vi "SetTensionVelocity.vi"(8 "error in (no error)":errorcluster, 11 "Tapedrive_ESP301 in":refnum<class "Tapedrive_ESP301.lvclass">) -> (0 "error out":errorcluster, 3 "Tapedrive_ESP301 out":refnum<class "Tapedrive_ESP301.lvclass">)   [LabVIEW 2013, in "Tapedrive_ESP301.lvclass"]
uses:
  Tapedrive_ESP301.lvclass
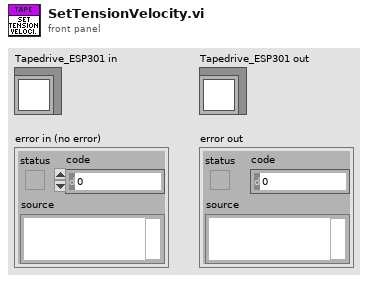
[diagram p1: front panel]
types:
  T1 = cluster{"Axis 1":cluster{"Value":dbl, "Min":dbl, "Max":dbl, "StepSize":dbl, "Tolerance":dbl, "ValueActual":dbl}, "Axis 2":cluster{"Value":dbl, "Min":dbl, "Max":dbl, "StepSize":dbl, "Tolerance":dbl, "ValueActual":dbl}}
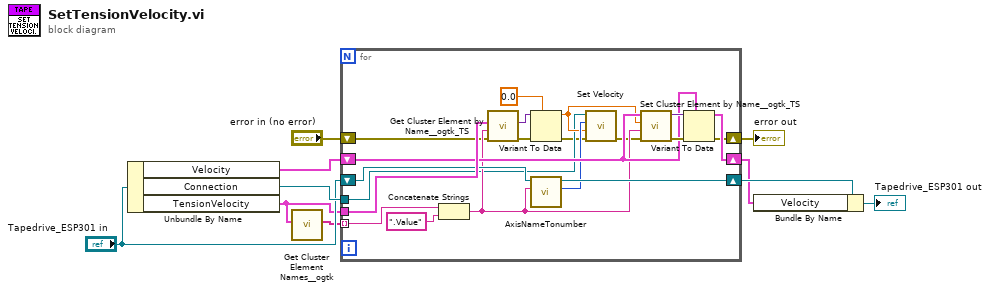
[diagram p0: block diagram]
diagram:
  n1 = Unbundle By Name("Tapedrive_ESP301 in") -> ("Velocity"=w10:T1, "Connection"=w5:refnum<visa-resource-name>, "TensionVelocity"=w2:T1)
  n2 = call <userlib>:"Get Cluster Element Names__ogtk.vi"("Cluster"=w2) -> ("Element Names"=w1:string[])  [unwired: 9 in, 1 out]
  n3 = for {
    tunnel: w1 -> [w30] mode=indexing
    tunnel: w2 -> [w28]
    shift-right: [w22] -> w3
    shift-left: w10 -> [w23]
    shift-right: [w20] -> w8
    shift-left: "Tapedrive_ESP301 in" -> [w21]
    tunnel: w5 -> [w16]
    shift-right: [w12] -> w7
    shift-left: "error in (no error)" -> [w11]
    n4 = Concatenate Strings(w30, ".Value" ("string")) -> (w19:string)
    n5 = call "Get Cluster Element by Name__ogtk_TS.vi"("error in (no error)"=w11, "Element Name"=w19, "Cluster"=w28) -> ("error out"=w15:errorcluster, "VElement"=w27:variant)  [unwired: 6 in, 1 out]
    n6 = Variant To Data(error in=w15, type=0.0, Variant=w27) -> (data=w17:dbl, error out=w14:errorcluster)
    n7 = call "AxisNameTonumber.vi"("Channel"=w19, "Tapedrive_ESP301 in"=w21) -> ("Axis No."=w18:i16, "Tapedrive_ESP301 out"=w20:refnum<class "Tapedrive_ESP301.lvclass">)  [unwired: 8 in]
    n8 = call <instrlib>:"Set Velocity.vi"("error in (no error)"=w14, "Velocity (units/s)"=w17, "Axis (1)"=w18, "VISA resource name"=w16) -> ("error out"=w13:errorcluster)  [unwired: 2 in, 1 out]
    n9 = call "Set Cluster Element by Name__ogtk_TS.vi"("error in (no error)"=w13, "Element Name (\"\": New Element Data Name)"=w19, "New Element Value"=w17, "Cluster"=w23) -> ("error out"=w25:errorcluster, "VCluster out"=w24:variant)  [unwired: 5 in, 1 out]
    n10 = Variant To Data(error in=w25, type=w23, Variant=w24) -> (data=w22:T1, error out=w12:errorcluster)
  }
  "error out" <- w7
  n11 = Bundle By Name(cluster=w8, "Velocity"=w3) -> (→"Tapedrive_ESP301 out":refnum<class "Tapedrive_ESP301.lvclass">)
